vi "RoadLaneDetection.vi"(0 "Color Plane (Color Plane Extraction 1)":i32(ring) items=["Red", "Green", "Blue", "Hue", "Saturation", "Luminance", "Value", "Intensity"], 7 "error in":errorcluster) -> (20 "Straight Edge (Find Straight Edge 1)":T2 {"Point2 (Real-World)"."Y" format="%.2f"; "Point2 (Real-World)"."X" format="%.2f"; "Point1 (Real-World)"."Y" format="%.2f"; "Point1 (Real-World)"."X" format="%.2f"; "Point2 (Pixels)"."Y" format="%.2f"; "Point2 (Pixels)"."X" format="%.2f"; "Point1 (Pixels)"."Y" format="%.2f"; "Point1 (Pixels)"."X" format="%.2f"}, 21 "Straight Edge (Find Straight Edge 2)":T2 {"Point2 (Real-World)"."Y" format="%.2f"; "Point2 (Real-World)"."X" format="%.2f"; "Point1 (Real-World)"."Y" format="%.2f"; "Point1 (Real-World)"."X" format="%.2f"; "Point2 (Pixels)"."Y" format="%.2f"; "Point2 (Pixels)"."X" format="%.2f"; "Point1 (Pixels)"."Y" format="%.2f"; "Point1 (Pixels)"."X" format="%.2f"}, 27 "error out":errorcluster)   [LabVIEW 2015]
uses:
  <vilib>/vision/Measure.llb/Straight Edge Options.ctl
  <vilib>/vision/Measure.llb/Straight Edge Process.ctl
  <vilib>/vision/Measure.llb/Edge Options.ctl
  <vilib>/vision/Measure.llb/Edge Polarity.ctl
  <vilib>/vision/NI_Vision_Development_Module.lvlib
panel:
  out "Image Out":T1(plugin-control)
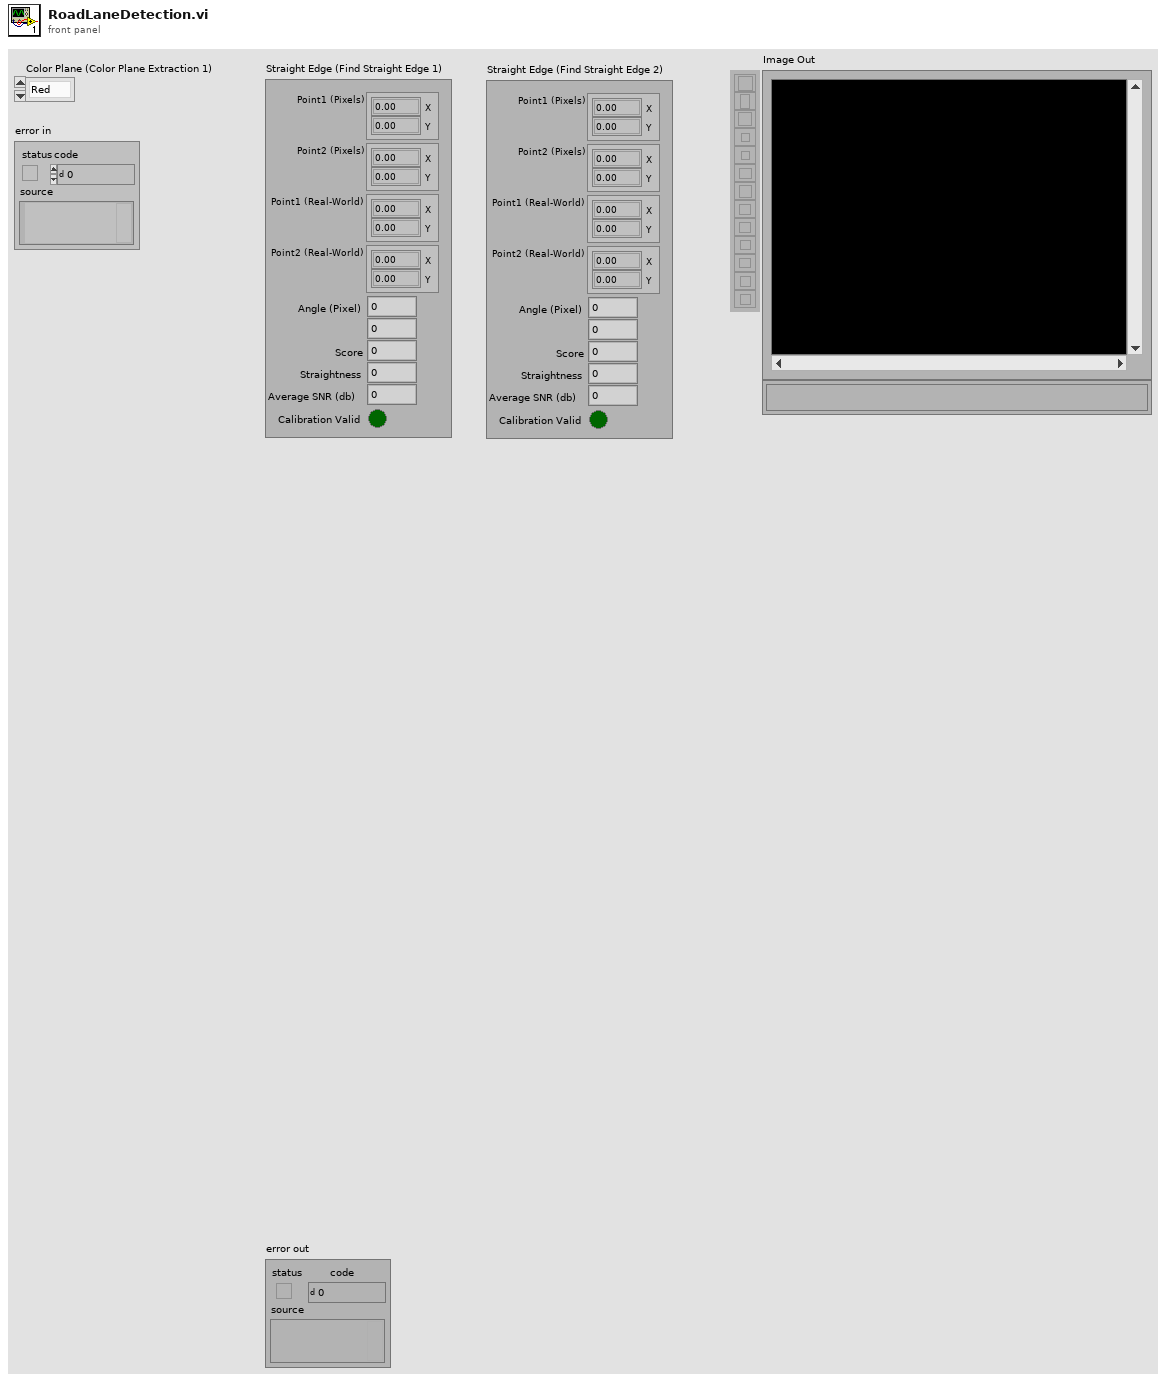
[diagram p1: front panel]
types:
  T1 = typedef "IMAQ Image.ctl" = refnum<image>
  T2 = cluster{"Point1 (Pixels)":cluster{"X":sgl, "Y":sgl}, "Point2 (Pixels)":cluster{"X":sgl, "Y":sgl}, "Point1 (Real-World)":cluster{"X":sgl, "Y":sgl}, "Point2 (Real-World)":cluster{"X":sgl, "Y":sgl}, "Angle (Pixel)":dbl, "Angle (Real-World)":dbl, "Score":dbl, "Straightness":dbl, "Average SNR (db)":dbl, "Calibration Valid":bool}
  T3 = typedef "Edge Options.ctl" = cluster{"Edge Polarity":T4, "Kernel Size":u32, "Width":u32, "Minimum Edge Strength":sgl, "Interpolation Type":enum32{"Zero Order", "Bilinear", "Quadratic", "Cubic", "Bilinear Fixed"}, "Data Processing Method":enum32{"Average", "Median"}}
  T4 = typedef "Edge Polarity.ctl" = u32
  T5 = cluster{"Search Direction":u32, "Edge Options":T3, "Show Search Area":bool, "Show Search Lines":bool, "Show Edges Found":bool, "Show Result":bool, "Search Area Color":u32, "Search Lines Color":u32, "Edge Locations Color":u32, "Result Color":u32, "Overlay Group Name":string}
  T6 = typedef "Straight Edge Options.ctl" = cluster{"Number of Lines":i32, "Type":T7, "Min. Score":dbl, "Max. Score":dbl, "Orientation":dbl, "Angle Range":dbl, "Angle Tolerance":dbl, "Step Size":u32, "Min. SNR (db)":dbl, "Min. Points (%)":dbl, "Hough Iterations":i32}
  T7 = typedef "Straight Edge Process.ctl" = enum32{"First Edge Rake", "Best Edge Rake", "Hough Edge Rake", "First Edge Projection", "Best Edge Projection"}
  T8 = cluster{"Global Rectangle":i32[], "Contours":cluster{"ID":enum32{"External", "Internal"}, "Type":u32, "Coordinates":i32[]}[]}
  T9 = typedef "Image Type" = u32
  T10 = cluster{"Point1 (Pixels)":cluster{"X":sgl, "Y":sgl}, "Point2 (Pixels)":cluster{"X":sgl, "Y":sgl}, "Point1 (Real-World)":cluster{"X":sgl, "Y":sgl}, "Point2 (Real-World)":cluster{"X":sgl, "Y":sgl}, "Angle (Pixel)":dbl, "Angle (Real-World)":dbl, "Score":dbl, "Straightness":dbl, "Average SNR (db)":dbl, "Calibration Valid":bool}[]
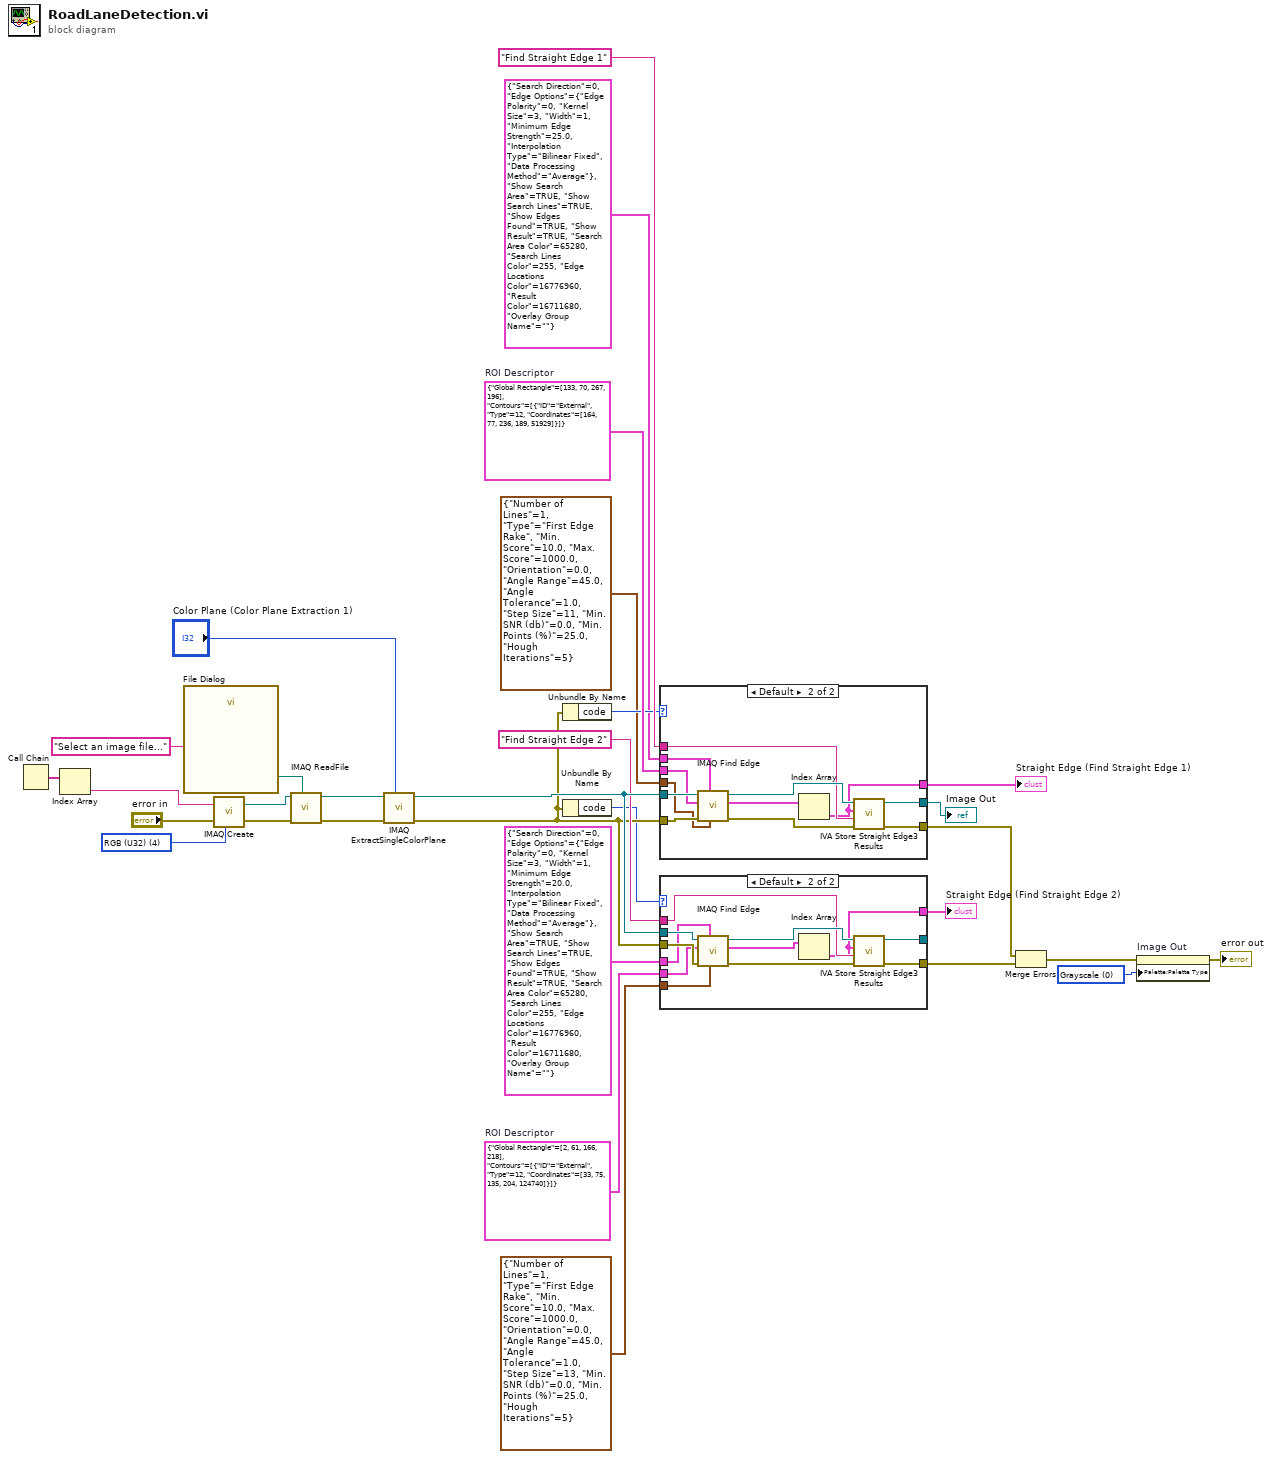
[diagram p0: block diagram]
diagram:
  w1 = u32 0 items=["Grayscale", "Binary", "Gradient", "Rainbow", "Temperature", "User Defined", "Binary 16 Bit", "Gradient 16 Bit", "Rainbow 16 Bit", "Temperature 16 Bit", "User Defined 16 Bit"] ("Palette Type")
  w13 = T8 {"Global Rectangle"=[2, 61, 166, 218], "Contours"=[{"ID"=enum."External", "Type"=12, "Coordinates"=[33, 75, 135, 204, 124740]}]}  # ROI Descriptor
  w20 = T8 {"Global Rectangle"=[133, 70, 267, 196], "Contours"=[{"ID"=enum."External", "Type"=12, "Coordinates"=[164, 77, 236, 189, 51929]}]}  # ROI Descriptor
  w24 = T9 4 items=["Grayscale (U8)", "Grayscale (I16)", "Grayscale (SGL)", "Complex (CSG)", "RGB (U32)", "HSL (U32)", "RGB (U64)", "Grayscale (U16)"] ("Image Type")
  n1 = Call Chain() -> (call chain=w28:string[])
  n2 = Index Array(array=w28) -> (element=w27:string)  [unwired: 1 in]
  n3 = call "File Dialog"("prompt"="Select an image file...") -> ("selected path"=w25:path)  [unwired: 6 in, 8 out]
  n4 = call "IMAQ Create"("Image Name"=w27, "Image Type"=w24, "error in (no error)"="error in") -> ("New Image"=w31:T1, "error out"=w30:errorcluster)  [unwired: 1 in, 1 out]
  n5 = call "IMAQ ReadFile"("File Path"=w25, "error in (no error)"=w30, "Image"=w31) -> ("error out"=w21:errorcluster, "Image Out"=w22:T1)  [unwired: 2 in, 5 out]
  n6 = call "IMAQ ExtractSingleColorPlane"("Color Plane"="Color Plane (Color Plane Extraction 1)", "error in (no error)"=w21, "Image Src"=w22) -> ("error out"=w11:errorcluster, "Image Dst Out"=w14:T1)  [unwired: 1 in, 6 out]
  n7 = Unbundle By Name(w11) -> ("code"=w18:i32)
  n8 = Unbundle By Name(w11) -> ("code"=w10:i32)
  n9 = case shown="Default" w18 {
    tunnel: w14 -> [w32 w44]
    tunnel: w11 -> [_ w43]
    tunnel: w20 -> [_ w37]
    tunnel: [w32 w41] -> w2
    tunnel: [_ w39] -> w6
    tunnel: "Find Straight Edge 1" ("Step Name") -> [_ w38]
    tunnel: T6 {"Number of Lines"=1, "Type"=enum."First Edge Rake", "Min. Score"=10.0, "Max. Score"=1000.0, "Orientation"=0.0, "Angle Range"=45.0, "Angle Tolerance"=1.0, "Step Size"=11, "Min. SNR (db)"=0.0, "Min. Points (%)"=25.0, "Hough Iterations"=5} ("Fit Options") -> [_ w36]
    tunnel: T5 {"Search Direction"=0, "Edge Options"={"Edge Polarity"=0, "Kernel Size"=3, "Width"=1, "Minimum Edge Strength"=25.0, "Interpolation Type"=enum."Bilinear Fixed", "Data Processing Method"=enum."Average"}, "Show Search Area"=TRUE, "Show Search Lines"=TRUE, "Show Edges Found"=TRUE, "Show Result"=TRUE, "Search Area Color"=65280, "Search Lines Color"=255, "Edge Locations Color"=16776960, "Result Color"=16711680, "Overlay Group Name"=""} ("Options") -> [_ w35]
    tunnel: [_ w33] -> w15
    frame -1074396199, -1074396198 {
      # "Discard Coordinate System Error"
    }
    frame Default {
      n10 = call "IMAQ Find Edge"("Line Fit Options"=w36, "Options"=w35, "error in (no error)"=w43, "ROI Descriptor"=w37, "Image"=w44) -> ("error out"=w40:errorcluster, "Straight Edges"=w34:T10, "Image Out"=w42:T1)  [unwired: 1 in, 3 out]
      n11 = Index Array(array=w34) -> (element=w33:T2)  [unwired: 1 in]
      n12 = call <vilib>:"IVA Store Straight Edge3 Results.vi"("error in (no error)"=w40, "Step Name"=w38, "Straight Edge"=w33, "Image in"=w42) -> ("error out"=w39:errorcluster, "Image dup"=w41:T1)  [unwired: 1 in, 5 out]
    }
  }
  "Straight Edge (Find Straight Edge 1)" <- w15
  "Image Out" <- w2
  n13 = case shown="Default" w10 {
    tunnel: w14 -> [w45 w57]
    tunnel: w11 -> [_ w56]
    tunnel: w13 -> [_ w50]
    tunnel: [w45 w54] -> _
    tunnel: [_ w52] -> w5
    tunnel: "Find Straight Edge 2" ("Step Name") -> [_ w51]
    tunnel: T6 {"Number of Lines"=1, "Type"=enum."First Edge Rake", "Min. Score"=10.0, "Max. Score"=1000.0, "Orientation"=0.0, "Angle Range"=45.0, "Angle Tolerance"=1.0, "Step Size"=13, "Min. SNR (db)"=0.0, "Min. Points (%)"=25.0, "Hough Iterations"=5} ("Fit Options") -> [_ w49]
    tunnel: T5 {"Search Direction"=0, "Edge Options"={"Edge Polarity"=0, "Kernel Size"=3, "Width"=1, "Minimum Edge Strength"=20.0, "Interpolation Type"=enum."Bilinear Fixed", "Data Processing Method"=enum."Average"}, "Show Search Area"=TRUE, "Show Search Lines"=TRUE, "Show Edges Found"=TRUE, "Show Result"=TRUE, "Search Area Color"=65280, "Search Lines Color"=255, "Edge Locations Color"=16776960, "Result Color"=16711680, "Overlay Group Name"=""} ("Options") -> [_ w48]
    tunnel: [_ w46] -> w7
    frame -1074396199, -1074396198 {
      # "Discard Coordinate System Error"
    }
    frame Default {
      n14 = call "IMAQ Find Edge"("Line Fit Options"=w49, "Options"=w48, "error in (no error)"=w56, "ROI Descriptor"=w50, "Image"=w57) -> ("error out"=w53:errorcluster, "Straight Edges"=w47:T10, "Image Out"=w55:T1)  [unwired: 1 in, 3 out]
      n15 = Index Array(array=w47) -> (element=w46:T2)  [unwired: 1 in]
      n16 = call <vilib>:"IVA Store Straight Edge3 Results.vi"("error in (no error)"=w53, "Step Name"=w51, "Straight Edge"=w46, "Image in"=w55) -> ("error out"=w52:errorcluster, "Image dup"=w54:T1)  [unwired: 1 in, 5 out]
    }
  }
  "Straight Edge (Find Straight Edge 2)" <- w7
  n17 = Merge Errors(w6, w5) -> (w4:errorcluster)
  n18 = property on="Image Out" class="ImageControl"(error in=w4, "Palette:Palette Type"=w1) -> (error out=→"error out":errorcluster)  [unwired: 1 in, 1 out]
